vi "get network adapter settings.vi"(8 "error in":errorcluster, 11 "system session in":refnum<k21>) -> (0 "error out":errorcluster, 1 "secondary network adapters":T1[](array[typedef]) {"IP address request mode" items=["Static"=1, "DHCP/Link Local"=2, "Link-Local Only"=4, "DHCP Only"=8]; "adapter type" items=["Ethernet"=1, "WLAN"=2]; "adapter mode" items=["Disabled"=1, "TCP/IP Ethernet"=2, "Deterministic"=4, "EtherCAT"=8, "TCP/IP WLAN Connect"=32, "TCP/IP WLAN Create"=64]}, 2 "primary network adapter":T1 {"IP address request mode" items=["Static"=1, "DHCP/Link Local"=2, "Link-Local Only"=4, "DHCP Only"=8]; "adapter type" items=["Ethernet"=1, "WLAN"=2]; "adapter mode" items=["Disabled"=1, "TCP/IP Ethernet"=2, "Deterministic"=4, "EtherCAT"=8, "TCP/IP WLAN Connect"=32, "TCP/IP WLAN Create"=64]}, 3 "system session out":refnum<k21>)   [LabVIEW 2016, in "SMI.lvlib" / "Controller.lvclass"]
uses:
  Controller.lvclass
  network adapter settings.ctl
  <vilib>/nisyscfg/Close (Hardware).vi
  <vilib>/nisyscfg/Find Hardware.vi
  <vilib>/nisyscfg/nisyscfg.lvlib
  <resource>/objmgr/niflexriosae.rc
  <resource>/objmgr/nicriosae.rc
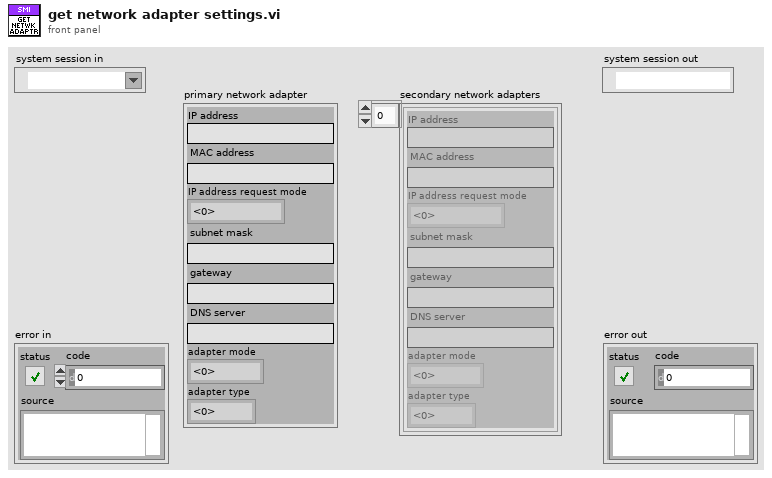
[diagram p1: front panel]
types:
  T1 = typedef "SMI.lvlib/Controller.lvclass/network adapter settings.ctl" = cluster{"IP address":string, "MAC address":string, "IP address request mode":u32, "subnet mask":string, "gateway":string, "DNS server":string, "adapter mode":u32, "adapter type":u32}
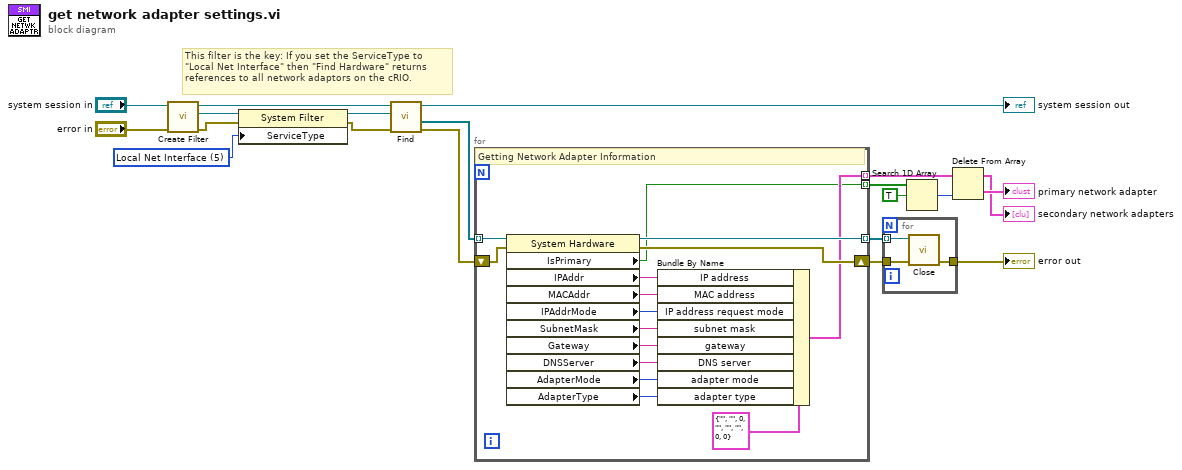
[diagram p0: block diagram]
diagram:
  w13 = u32 5 items=["NI Network Resource", "NI Real-Time", "NI System Configuration", "NI Web Interface", "Local System", "Local Net Interface", "Local Time Keeper", "Local Time Reference", "LXI Instrument"] ("Service Type")
  # "This filter is the key: If you set the ServiceType to\n\"Local Net Interface\" then \"Find Hardware\" returns\nreferences to all network adaptors on the cRIO."
  n1 = call <vilib>:"Create Filter.vi"("error in (no error)"="error in", "Session in"="system session in") -> ("error out"=w16:errorcluster, "Filter out"=w12:refnum<k20>, "Session out"=w11:refnum<k21>)  [unwired: 7 in]
  n2 = property class="System Filter"(reference=w12, error in=w16, "ServiceType"=w13) -> (reference out=w14:refnum<k20>, error out=w15:errorcluster)
  n3 = call-poly <vilib>:"Find.vi"("error in (no error)"=w15, "Filter in"=w14, "Session in"=w11) -> ("error out"=w17:errorcluster, "Resources out"=w7:refnum<k20>[], "Session out"=→"system session out":refnum<k21>)  [unwired: 5 in, 1 out]
  n4 = for {
    tunnel: w7 -> [w34] mode=indexing
    shift-right: [w23] -> w20
    shift-left: w17 -> [w35]
    tunnel: [w29] -> w10 mode=indexing
    tunnel: [w22] -> w6 mode=indexing
    tunnel: [w21] -> w5 mode=indexing
    # "Getting Network Adapter Information"
    n5 = property class="System Hardware"(reference=w34, error in=w35) -> (reference out=w29:refnum<k20>, error out=w23:errorcluster, "IsPrimary"=w21:bool, "IPAddr"=w24:string, "MACAddr"=w30:string, "IPAddrMode"=w27:u32, "SubnetMask"=w31:string, "Gateway"=w32:string, "DNSServer"=w33:string, "AdapterMode"=w26:u32, "AdapterType"=w25:u32)
    n6 = Bundle By Name(cluster=T1 {"IP address"="", "MAC address"="", "IP address request mode"=0, "subnet mask"="", "gateway"="", "DNS server"="", "adapter mode"=0, "adapter type"=0} ("Network Adapter Settings"), "IP address"=w24, "MAC address"=w30, "IP address request mode"=w27, "subnet mask"=w31, "gateway"=w32, "DNS server"=w33, "adapter mode"=w26, "adapter type"=w25) -> (w22:T1)
  }
  n7 = for {
    tunnel: [w38] -> w19
    tunnel: w20 -> [w37]
    tunnel: w10 -> [w36] mode=indexing
    n8 = call-poly <vilib>:"Close.vi"("error in (no error)"=w37, "Resource in"=w36) -> ("error out"=w38:errorcluster)  [unwired: 9 in]
  }
  "error out" <- w19
  n9 = Search 1D Array(1D array=w5, element=TRUE) -> (index of element=w3:i32)  [unwired: 1 in]
  n10 = Delete From Array(array=w6, index=w3) -> (deleted portion=→"primary network adapter":T1, array with subset deleted=→"secondary network adapters":T1[])  [unwired: 1 in]
